vi "Get All Possible Connections.vi"(8 "error in (no error)":errorcluster, 11 "Hardware Ref in":T2 format="%.0x") -> (0 "error out":errorcluster, 2 "Possible Connections":T1[](array[typedef]), 3 "Hardware Ref out":T2 format="%.0x", 4 "Found?":bool)   [LabVIEW 2017, in "Routing and Faulting Hardware API.lvlib"]
uses:
  Routing and Faulting Hardware API.lvlib
  <vilib>/NI Veristand/Custom Device API/Custom Device Item Ref.ctl
  Types/Possible Connections for Endpoint.ctl
  <vilib>/NI Veristand/Custom Device API/Custom Device API.lvlib
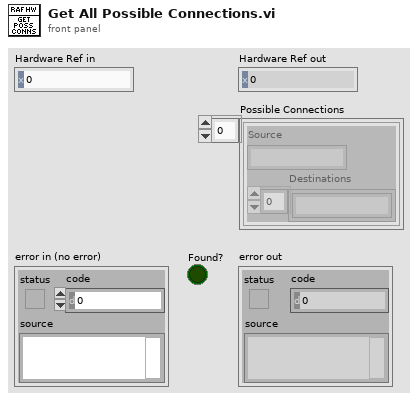
[diagram p1: front panel]
types:
  T1 = typedef "Routing and Faulting Hardware API.lvlib/Possible Connections for Endpoint.ctl" = cluster{"Source":string, "Destinations":string[]}
  T2 = typedef "Custom Device API.lvlib/Custom Device Item Ref.ctl" = u64
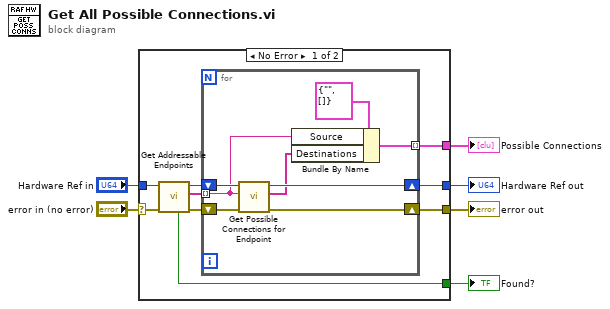
[diagram p0: block diagram]
diagram:
  n1 = case shown="No Error" "error in (no error)" {
    selector: "error in (no error)" -> [w15 w25]
    tunnel: [w8 w25] -> w6
    tunnel: "Hardware Ref in" -> [w14 w24]
    tunnel: [w11 w24] -> w3
    tunnel: [w9 _] -> w2
    tunnel: [w7 _] -> w1
    frame No Error {
      n2 = call "Get Addressable Endpoints.vi"("error in (no error)"=w15, "Hardware Ref in"=w14) -> ("error out"=w13:errorcluster, "Addressable Endpoints"=w10:string[], "Hardware Ref out"=w12:T2, "Found?"=w7:bool)  [unwired: 6 in]
      n3 = for {
        shift-right: [w22] -> w8
        shift-left: w13 -> [w23]
        shift-right: [w20] -> w11
        shift-left: w12 -> [w21]
        tunnel: w10 -> [w18] mode=indexing
        tunnel: [w16] -> w9 mode=indexing
        n4 = call "Get Possible Connections for Endpoint.vi"("error in (no error)"=w23, "Endpoint"=w18, "Hardware Ref in"=w21) -> ("error out"=w22:errorcluster, "Possible Connections"=w17:string[], "Hardware Ref out"=w20:T2)  [unwired: 6 in]
        n5 = Bundle By Name(cluster=T1 {"Source"="", "Destinations"=[]} ("Possible Connections for Endpoint"), "Source"=w18, "Destinations"=w17) -> (w16:T1)
      }
    }
    frame Error {
    }
  }
  "Hardware Ref out" <- w3
  "error out" <- w6
  "Possible Connections" <- w2
  "Found?" <- w1
